vi "LJM_ByteArrayToINT32.vi"(1 "Byte Array":u8[](array[numeric])) -> (0 "I32":i32)   [LabVIEW 2020]
panel:
  # "Converts the first 4 elements of a big-endian byte array to a I32"
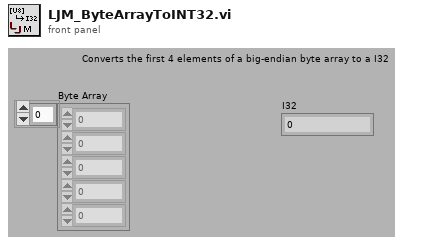
[diagram p1: front panel]
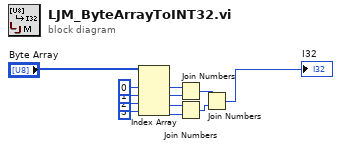
[diagram p0: block diagram]
diagram:
  n1 = Index Array(array="Byte Array", index #1=0 ("Index"), index #2=1 ("Index"), index #3=2 ("Index"), index #4=3 ("Index")) -> (element #1=w8:u8, element #2=w9:u8, element #3=w5:u8, element #4=w4:u8)
  n2 = Join Numbers(hi=w8, lo=w9) -> ((hi.lo)=w2:u16)
  n3 = Join Numbers(hi=w5, lo=w4) -> ((hi.lo)=w3:u16)
  n4 = Join Numbers(hi=w2, lo=w3) -> ((hi.lo)=→"I32":u32)
